vi "弹窗-自定义导出.vi"() -> ()   [LabVIEW 2017]
panel:
  out "导出条件引用":refnum<vi>
  out "导出条件":T1
  in  "选项卡控件":enum32{"定时配置", "自定义导出"}(tab)
  out "下个累积时刻":string
  in  "配置自动导出":bool
  out "下个导出时刻":string caption="下个自动导出时刻"
  in  "起始":timestamp caption="起始 (包含)" format="%<%x %X>T"
  in  "截止":timestamp caption="截止 (不含)" format="%<%x %X>T"
  in  "范围选项":enum16{"自定义", "本月", "上月"}(ring)=enum."上月" caption="预设选项"
  in  "导出":bool
  in  "独立导出?":bool
  out "手动导出提示语":string
  in  "取消":bool
  out "信号-关闭窗口":bool=TRUE
  # "时间范围设定"
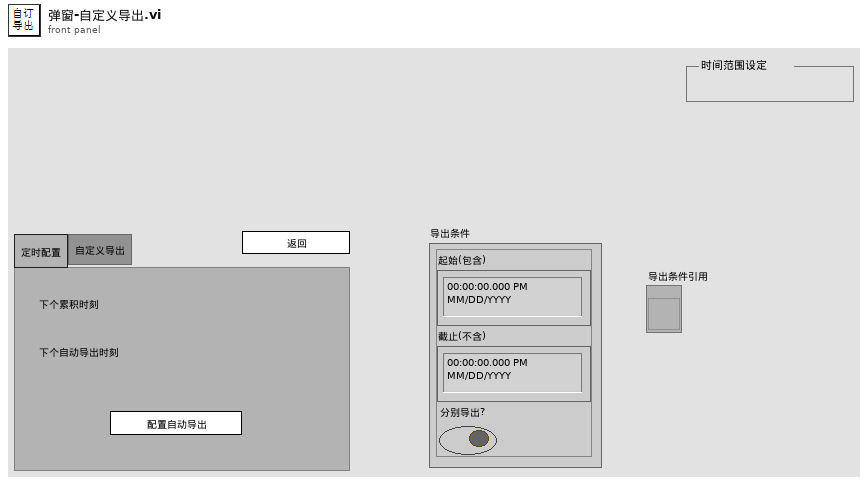
[diagram p1: front panel]
types:
  T1 = typedef "文件导出条件.ctl" = cluster{"起始(包含)":timestamp, "截止(不含)":timestamp, "分别导出?":bool}
  T2 = enum32{"Invalid", "Standard", "Closed", "Hidden", "Minimized", "Maximized"}
  T3 = typedef "簇-输入.ctl" = cluster{"配置文件动作":T4, "数据输入":variant}
  T4 = typedef "枚举-配置文件动作.ctl" = enum16{"初始化加载配置", "读取配置", "写入-屏幕键盘", "写入-静音延迟", "写入-主要探头类型", "写入-串口配置", "写入-累积定时", "写入-导出定时", "保存配置到文件"}
  T5 = typedef "定时配置.ctl" = cluster{"定时模式":enum16{"绝对时间", "相对时间"}, "单位":enum16{"年", "月", "日", "时", "分"}, "间隔":u8, "目标时刻":timestamp}
  T6 = typedef "簇-配置文件内容.ctl" = cluster{"调试模式？":bool, "屏幕键盘？":bool, "软件版本":string, "静音延迟 s":u16, "主要探头类型":T7, "串口配置":cluster{"COM口":refnum<visa-resource-name>, "波特率":enum16{"9600", "19200"}, "读写超时ms":i16, "丢包判定次数":i16}, "定时配置-累积分段":T8, "定时配置-自动导出":cluster{"定时配置-自动导出":T8, "分别导出?":bool}}
  T7 = typedef "枚举-主要探头类型.ctl" = enum16{"网络探头", "串口探头"}
  T8 = typedef "簇-定时配置.ctl" = cluster{"定时模式":enum16{"绝对时间", "相对时间"}, "单位":enum16{"年", "月", "日", "时", "分"}, "间隔":u8, "目标时刻":timestamp}
  T9 = typedef "LVDateTimeRec.ctl" = cluster{"秒数的小数部分":dbl, "秒":i32, "分":i32, "时":i32, "日":i32, "月":i32, "年":i32, "天数（周）":i32, "天数（年）":i32, "DST":i32}
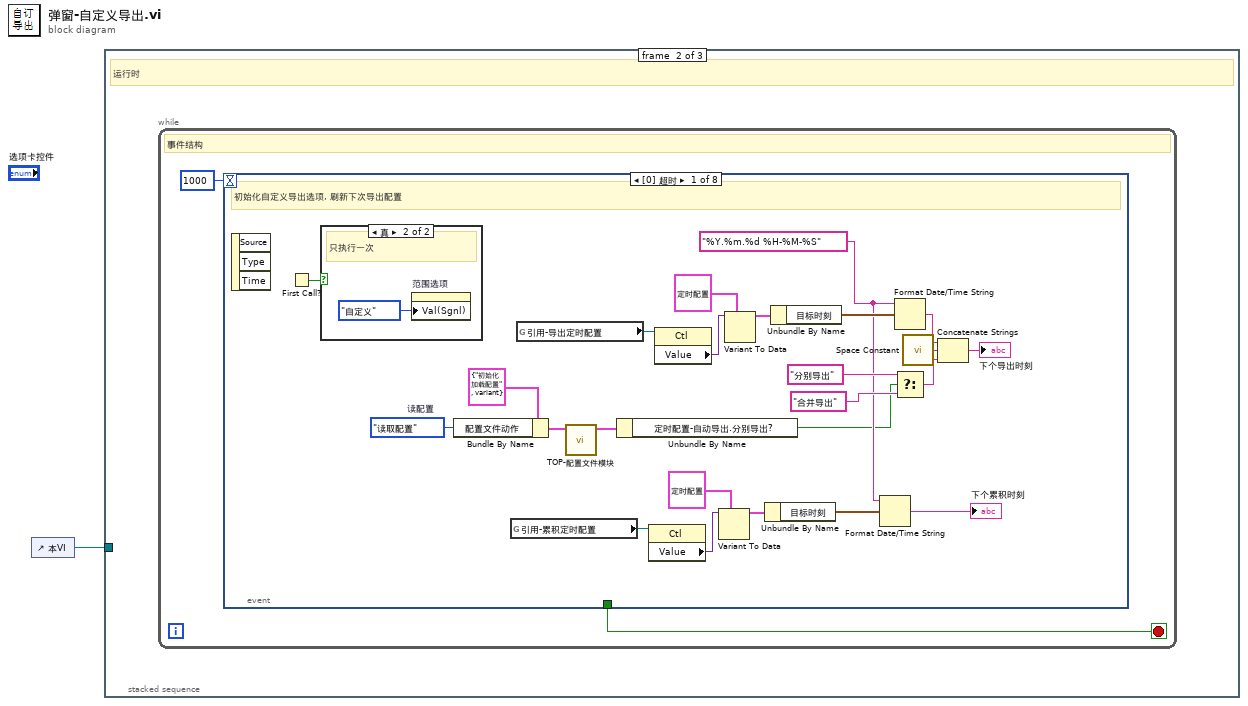
[diagram p0: block diagram]
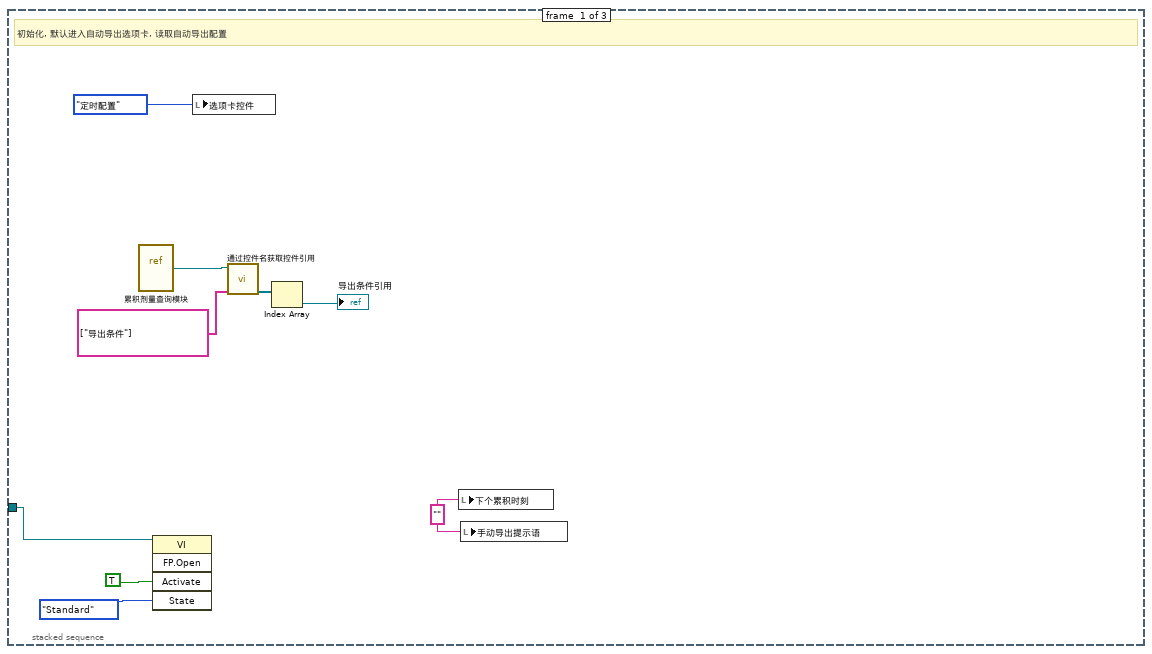
[diagram p2: hidden frame]
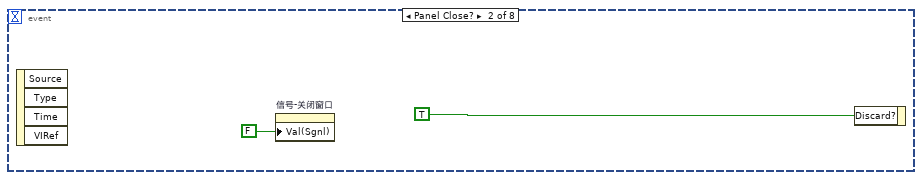
[diagram p4: hidden frame]
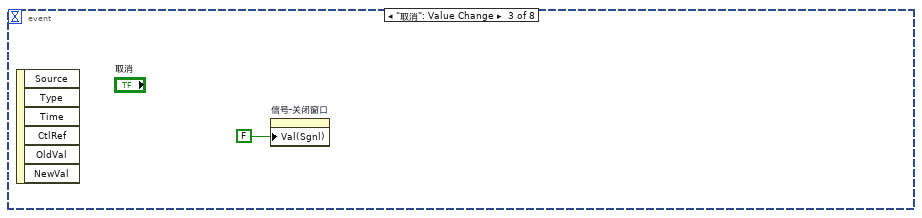
[diagram p5: hidden frame]
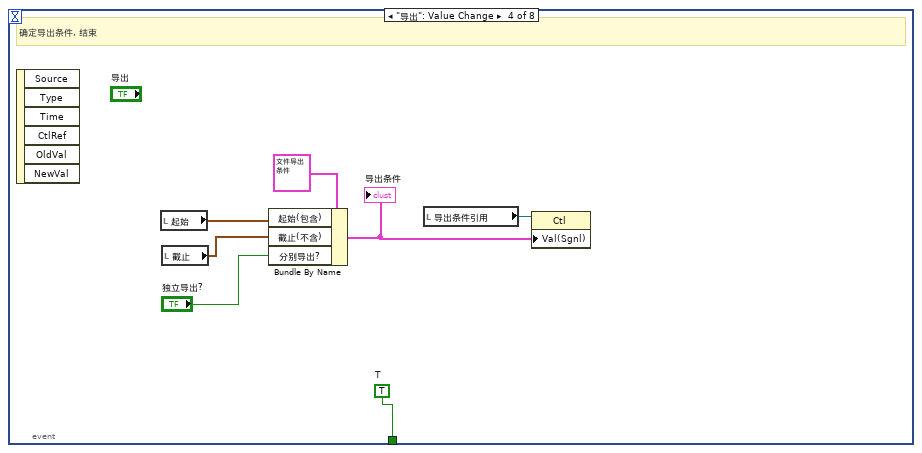
[diagram p6: hidden frame]
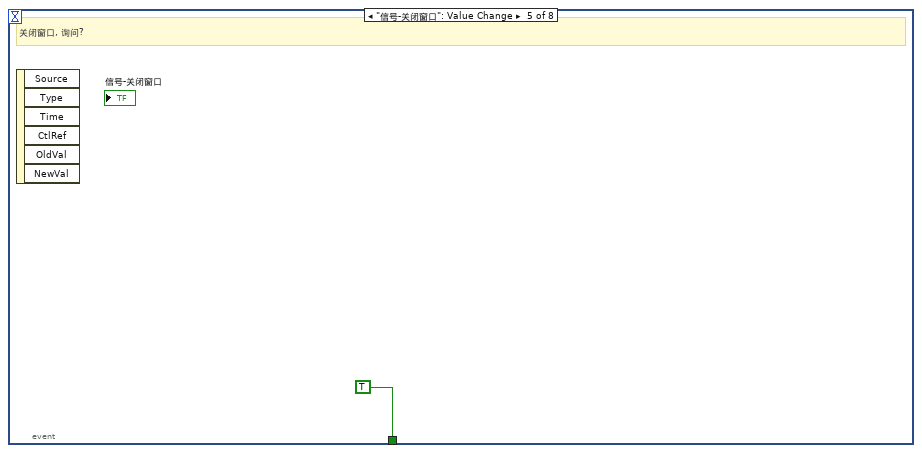
[diagram p7: hidden frame]
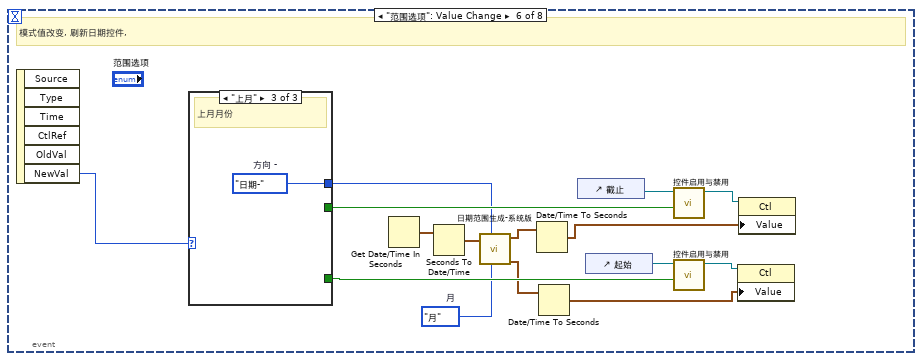
[diagram p8: hidden frame]
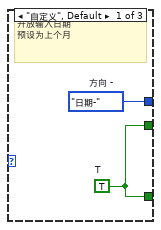
[diagram p9: hidden frame]
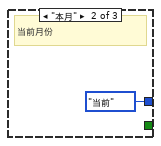
[diagram p10: hidden frame]
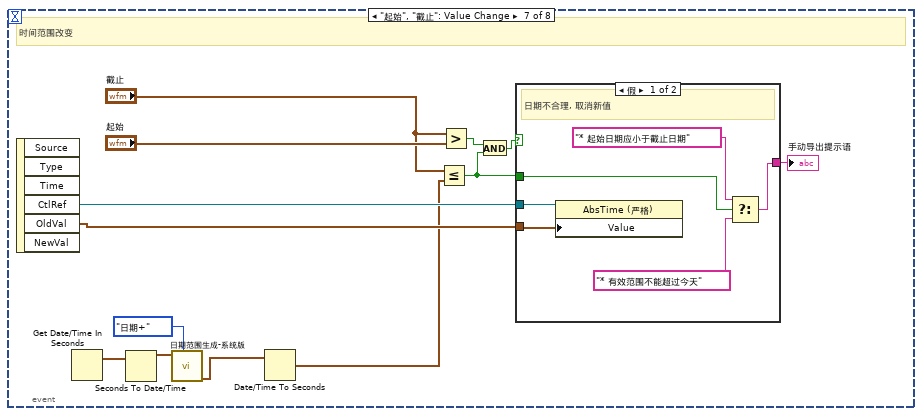
[diagram p11: hidden frame]
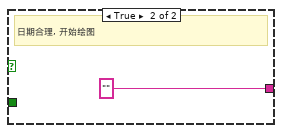
[diagram p12: hidden frame]
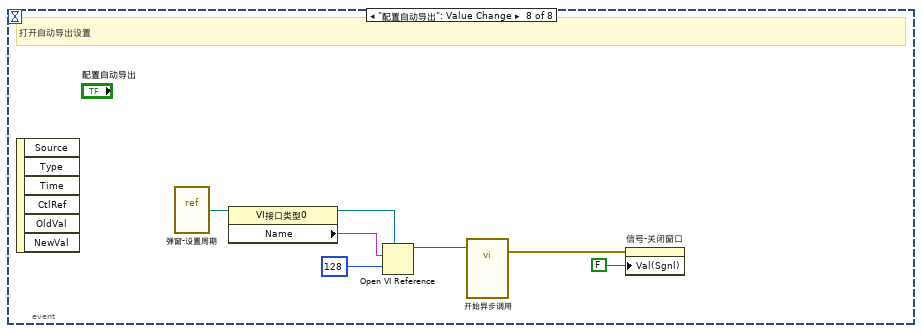
[diagram p13: hidden frame]
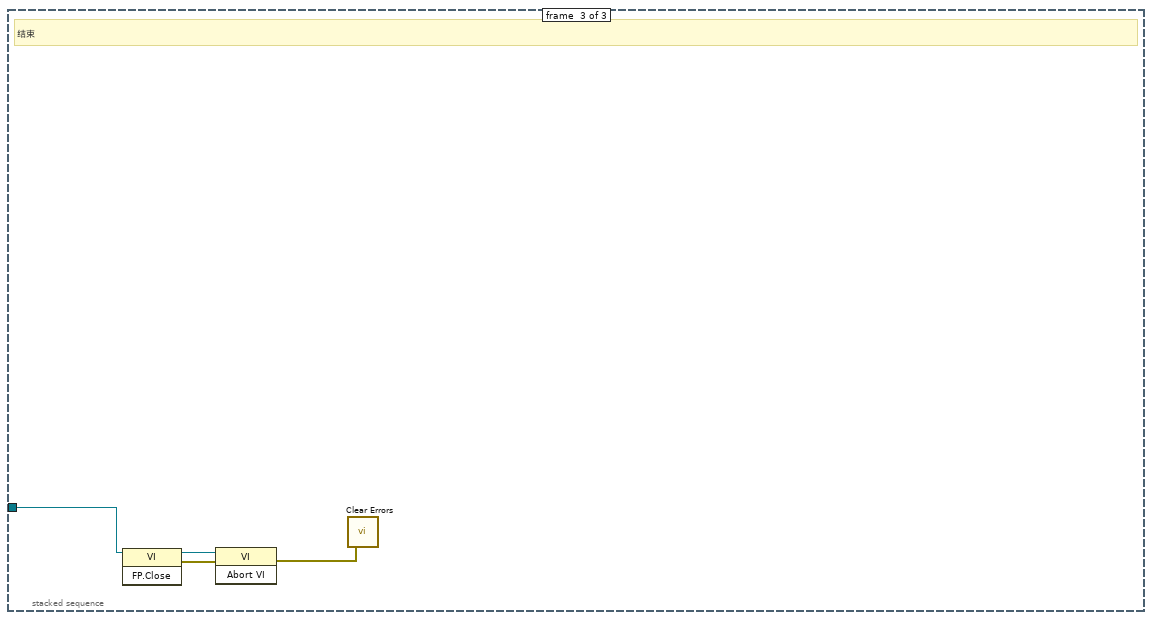
[diagram p14: hidden frame]
diagram:
  n1 = control-ref of="本VI"() -> (w1:refnum<vi>)
  n2 = stacked-sequence {
    tunnel: w1 -> [w10 _ w98]
    frame #0 {
      w6 = "" ("手动导出提示语")
      # "初始化, 默认进入自动导出选项卡, 读取自动导出配置"
      n3 = vi-ref "累积剂量查询模块.vi"() -> (w4:refnum<vi>)
      n4 = invoke class="VI" method="FP.Open"(reference=w10, "Activate"=TRUE ("激活？"), "State"=T2."Standard" ("状态")) -> ()  [unwired: 2 in, 5 out]
      n5 = local write "选项卡控件"(enum32{"定时配置", "自定义导出"}."定时配置" ("选项卡控件")) -> ()
      n6 = call "通过控件名获取控件引用.vi"("控件名数组"=string[] ["导出条件"], "VI引用"=w4) -> ("控件引用输出"=w5:refnum<vi>[])  [unwired: 7 in, 2 out]
      n7 = Index Array(array=w5) -> (element=→"导出条件引用":refnum<vi>)  [unwired: 1 in]
      n8 = local write "下个累积时刻"(w6) -> ()
      n9 = local write "手动导出提示语"(w6) -> ()
    }
    frame #1 {
      # "运行时"
      n10 = while {
        stop <- w12 stop-if-true
        # "事件结构"
        n11 = event shown="[0] 超时" {
          selector: _ -> [_ _ _ _ _ _ _ _]
          dyn-events: _ -> [_ _ _ _ _ _ _ _]
          timeout: 1000 -> [_ _ _ _ _ _ _ _]
          tunnel: [_ _ _ w45 TRUE _ _ _] -> w12
          event Timeout {
            w14 = 枚举-配置文件动作."读取配置"  # 读配置
            w19 = "%Y.%m.%d %H-%M-%S" ("时间格式字符串(%c)")
            # "初始化自定义导出选项, 刷新下次导出配置"
            n12 = event-data() -> ()  [unwired: 1 in, 3 out]
            n13 = First Call?() -> (First Call?: T/F=w36:bool)
            n14 = case shown="真" w36 {
              frame False {
              }
              frame True {
                # "只执行一次"
                n15 = property on="范围选项" class="Enum (严格)"("Val(Sgnl)"=enum16{"自定义", "本月", "上月"}."自定义" ("值(信号)")) -> ()  [unwired: 2 in, 2 out]
              }
            }
            n16 = Bundle By Name(cluster=T3 {"配置文件动作"=enum."初始化加载配置", "数据输入"=variant} ("输入"), "配置文件动作"=w14) -> (w17:T3)
            n17 = global read "全局变量-35点监测.vi" "引用-累积定时配置"() -> (w21:refnum<vi>)
            n18 = global read "全局变量-35点监测.vi" "引用-导出定时配置"() -> (w35:refnum<vi>)
            n19 = call "TOP-配置文件模块.vi"("输入"=w17) -> ("配置文件"=w16:T6)  [unwired: 9 in, 1 out]
            n20 = Unbundle By Name(w16) -> ("定时配置-自动导出.分别导出?"=w13:bool)
            n21 = property class="Ctl"(reference=w21) -> ("Value"=w22:variant)  [unwired: 1 in, 2 out]
            n22 = property class="Ctl"(reference=w35) -> ("Value"=w34:variant)  [unwired: 1 in, 2 out]
            n23 = Variant To Data(type=T5 {"定时模式"=enum."绝对时间", "单位"=enum."年", "间隔"=0, "目标时刻"=timestamp(0 s since 1904-01-01)} ("定时配置"), Variant=w22) -> (data=w23:T5)  [unwired: 1 in, 1 out]
            n24 = Variant To Data(type=T5 {"定时模式"=enum."绝对时间", "单位"=enum."年", "间隔"=0, "目标时刻"=timestamp(0 s since 1904-01-01)} ("定时配置"), Variant=w34) -> (data=w33:T5)  [unwired: 1 in, 1 out]
            n25 = Unbundle By Name(w23) -> ("目标时刻"=w20:timestamp)
            n26 = Unbundle By Name(w33) -> ("目标时刻"=w32:timestamp)
            n27 = Format Date/Time String(time format string (%c)=w19, seconds (now)=w20) -> (date/time string=→"下个累积时刻":string)  [unwired: 1 in]
            n28 = Format Date/Time String(time format string (%c)=w19, seconds (now)=w32) -> (date/time string=w31:string)  [unwired: 1 in]
            n29 = Select(t="分别导出" ("时间格式字符串(%c)"), s=w13, f="合并导出" ("时间格式字符串(%c)")) -> (s? t:f=w30:string)
            n30 = call <vilib>:"Space Constant.vi"() -> ("String"=w28:string)
            n31 = Concatenate Strings(w31, w28, w30) -> (→"下个导出时刻":string)
          }
          event Panel Close? {
            n32 = event-data() -> ()  [unwired: 1 in, 4 out]
            n33 = property on="信号-关闭窗口" class="Bool (严格)"("Val(Sgnl)"=FALSE ("值(信号)")) -> ()  [unwired: 2 in, 2 out]
            n34 = event-data("Discard?"=TRUE ("放弃？")) -> ()  [unwired: 1 in, 1 out]
          }
          event "取消": Value Change {
            n35 = event-data() -> ()  [unwired: 1 in, 6 out]
            n36 = property on="信号-关闭窗口" class="Bool (严格)"("Val(Sgnl)"=FALSE ("值(信号)")) -> ()  [unwired: 2 in, 2 out]
          }
          event "导出": Value Change {
            w45 = TRUE  # T
            # "确定导出条件, 结束"
            n37 = event-data() -> ()  [unwired: 1 in, 6 out]
            n38 = local read "起始"() -> (w44:timestamp)
            n39 = local read "截止"() -> (w43:timestamp)
            n40 = Bundle By Name(cluster=T1 {"起始(包含)"=timestamp(0 s since 1904-01-01), "截止(不含)"=timestamp(0 s since 1904-01-01), "分别导出?"=FALSE} ("导出条件"), "起始(包含)"=w44, "截止(不含)"=w43, "分别导出?"="独立导出?") -> (w42:T1)
            "导出条件" <- w42
            n41 = local read "导出条件引用"() -> (w41:refnum<vi>)
            n42 = property class="Ctl"(reference=w41, "Val(Sgnl)"=w42) -> ()  [unwired: 1 in, 2 out]
          }
          event "信号-关闭窗口": Value Change {
            # "关闭窗口, 询问?"
            n43 = event-data() -> ()  [unwired: 1 in, 6 out]
          }
          event "范围选项": Value Change {
            w54 = enum16{"年", "月", "日", "时", "分"}."月"  # 月
            # "模式值改变, 刷新日期控件,"
            n44 = event-data() -> ("NewVal"=w63:enum16{"自定义", "本月", "上月"})  [unwired: 1 in, 5 out]
            n45 = case shown="\"上月\"" w63 {
              tunnel: [w65 _ _] -> w62
              tunnel: [w65 _ _] -> w61
              tunnel: [w64 enum16{"当前", "日期+", "日期-"}."当前" ("方向 -") w67] -> w49
              frame "自定义", Default {
                w64 = enum16{"当前", "日期+", "日期-"}."日期-"  # 方向 -
                w65 = TRUE  # T
                # "开放输入日期\n预设为上个月"
              }
              frame "本月" {
                # "当前月份"
              }
              frame "上月" {
                w67 = enum16{"当前", "日期+", "日期-"}."日期-"  # 方向 -
                # "上月月份"
              }
            }
            n46 = Get Date/Time In Seconds() -> (seconds since 1Jan1904=w58:timestamp)
            n47 = Seconds To Date/Time(time stamp (now)=w58) -> (date time rec=w57:T9)  [unwired: 1 in]
            n48 = call "日期范围生成-系统版.vi"("单位"=w54, "方向"=w49, "日期时间记录"=w57) -> ("下限"=w55:T9, "上限"=w56:T9)  [unwired: 7 in]
            n49 = Date/Time To Seconds(2:w56) -> (0:w51:timestamp)  [unwired: 1 in]
            n50 = Date/Time To Seconds(2:w55) -> (0:w50:timestamp)  [unwired: 1 in]
            n51 = control-ref of="截止"() -> (w53:refnum<vi>)
            n52 = control-ref of="起始"() -> (w52:refnum<vi>)
            n53 = call "控件启用与禁用.vi"("启用？"=w62, "控件引用"=w53) -> ("引用输出"=w60:refnum<vi>)  [unwired: 9 in]
            n54 = call "控件启用与禁用.vi"("启用？"=w61, "控件引用"=w52) -> ("引用输出"=w59:refnum<vi>)  [unwired: 9 in]
            n55 = property class="Ctl"(reference=w59, "Value"=w50) -> ()  [unwired: 1 in, 2 out]
            n56 = property class="Ctl"(reference=w60, "Value"=w51) -> ()  [unwired: 1 in, 2 out]
          }
          event "起始", "截止": Value Change {
            # "时间范围改变"
            n57 = event-data() -> ("CtlRef"=w79:refnum<vi>, "OldVal"=w78:timestamp)  [unwired: 1 in, 4 out]
            n58 = Get Date/Time In Seconds() -> (seconds since 1Jan1904=w75:timestamp)
            n59 = Seconds To Date/Time(time stamp (now)=w75) -> (date time rec=w74:T9)  [unwired: 1 in]
            n60 = call "日期范围生成-系统版.vi"("方向"=enum16{"当前", "日期+", "日期-"}."日期+", "日期时间记录"=w74) -> ("下限"=w69:T9)  [unwired: 8 in, 1 out]
            n61 = Date/Time To Seconds(2:w69) -> (0:w72:timestamp)  [unwired: 1 in]
            n62 = Less Or Equal?(x="截止", y=w72) -> (x <= y?=w70:bool)
            n63 = Greater?(x="截止", y="起始") -> (0:w80:bool)
            n64 = And(x=w80, y=w70) -> (x .and. y?=w71:bool)
            n65 = case shown="假" w71 {
              tunnel: w79 -> [w86 _]
              tunnel: w78 -> [w85 _]
              tunnel: [w83 ""] -> w77
              tunnel: w70 -> [w84 _]
              frame False {
                # "日期不合理, 取消新值"
                n66 = property class="AbsTime (严格)"(reference=w86, "Value"=w85) -> ()  [unwired: 1 in, 2 out]
                n67 = Select(t="* 起始日期应小于截止日期", s=w84, f="* 有效范围不能超过今天") -> (s? t:f=w83:string)
              }
              frame True {
                # "日期合理, 开始绘图"
              }
            }
            "手动导出提示语" <- w77
          }
          event "配置自动导出": Value Change {
            # "打开自动导出设置"
            n68 = event-data() -> ()  [unwired: 1 in, 6 out]
            n69 = vi-ref "弹窗-设置周期.vi"() -> (w92:refnum<vi>)
            n70 = property class="VI接口类型0"(reference=w92) -> (reference out=w88:refnum<vi>, "Name"=w94:string)  [unwired: 1 in, 1 out]
            n71 = Open VI Reference(type specifier VI Refnum (for type only)=w88, vi path=w94, options=128 ("选项")) -> (vi reference=w91:refnum<vi>)  [unwired: 3 in, 1 out]
            n72 = call-by-ref "开始异步调用"(reference=w91) -> (error out=w89:errorcluster)  [unwired: 13 in, 1 out]
            n73 = property on="信号-关闭窗口" class="Bool (严格)"(error in=w89, "Val(Sgnl)"=FALSE ("值(信号)")) -> ()  [unwired: 1 in, 2 out]
          }
        }
      }
    }
    frame #2 {
      # "结束"
      n74 = invoke class="VI" method="FP.Close"(reference=w98) -> (reference out=w97:refnum<vi>, error out=w96:errorcluster)  [unwired: 2 in, 1 out]
      n75 = invoke class="VI" method="Abort VI"(reference=w97, error in=w96) -> (error out=w95:errorcluster)  [unwired: 1 in, 2 out]
      n76 = call <vilib>:"Clear Errors.vi"("error in (no error)"=w95) -> ()  [unwired: 5 in, 2 out]
    }
  }
